vi "ADXL345 I2C Accelerometer.vi"() -> ()   [LabVIEW 2025]
doc: "ADXL345 I2C Accelerometer\n\nThis example shows how to use the ADXL 345 Accelerometer sensor connected to I2C.\n\nThis example expects a USB cable connected from your development PC to the Type B USB Jack (next to the power input) on the roboRIO."
uses:
  <vilib>/Rock Robotics/SystemInterfaces/i2clib/i2c_bus.ctl
  <vilib>/Rock Robotics/WPI/Accelerometer/WPI_AccelerometerADXL345 Axes.ctl
  <vilib>/Rock Robotics/WPI/Accelerometer/ADXL345 Range.ctl
  <vilib>/Rock Robotics/WPI/Accelerometer/WPI_AccelerometerADXL345_I2C_Open.vi
panel:
  out "Z Acceleration":dbl
  out "Y Acceleration":dbl
  in  "Accel Range":T1 items=["+/- 2 g", "+/- 4 g", "+/- 8 g", "+/- 16 g"]
  in  "ADXL345 Axes":T2={"X-Axis"=TRUE, "Y-Axis"=FALSE, "Z-Axis"=FALSE}
  in  "I2C Bus":T3
  out "X Acceleration":dbl
  out "error out":errorcluster
  in  "stop":bool
  # "Set these inputs before running."
  # "Output information"
  # "This shows wiring for the ADXL345 accelerometer on a common sparkfun breakout board."
  # "ADXL345\nGND (black wire)-----\nVCC (red wire)--------\nSCL (yellow wire)-----\nSDA (white wire)------"
  # "roboRIO\nI2C  \nI2C   3.3V\nI2C   SCL\nI2C   SDA"
  # "This shows wiring for the ADXL345 accelerometer on a common kit of parts breakout board.\nNote the I2C header provides 3.3V, so this sensor gets its 5V power from the 5V rail - in this case DIO-0."
  # "ADXL345\n0V (black wire)--------\n5V (red wire)----------\nSCL (yellow wire)-----\nSDA (white wire)------"
  # "roboRIO\nI2C  \nDIO-0  V\nI2C   SCL\nI2C   SDA"
  # "accelerometer"
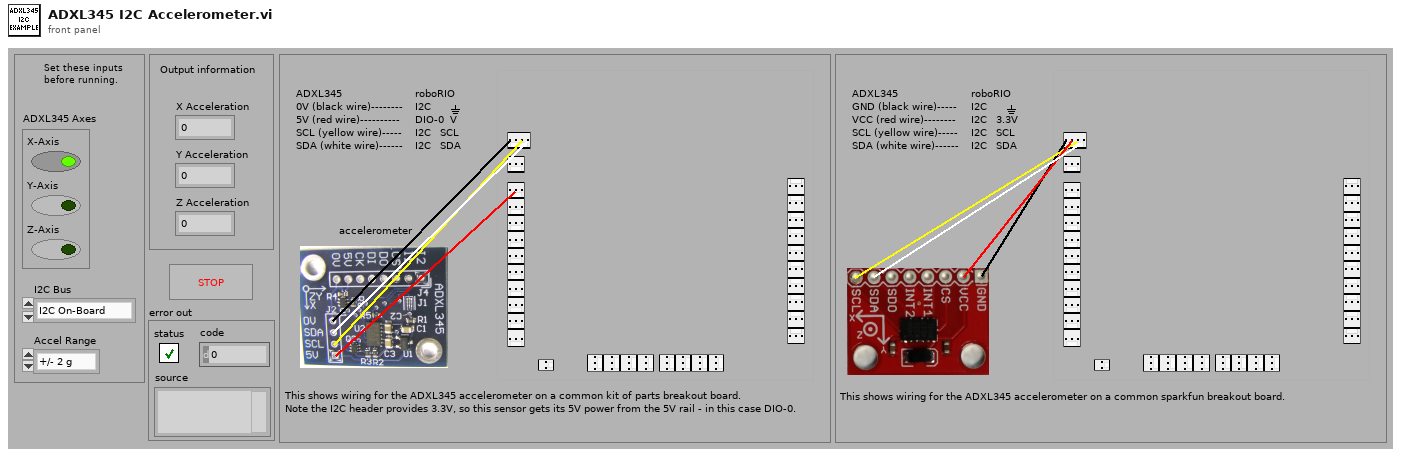
[diagram p1: front panel]
types:
  T1 = typedef "ADXL345 Range.ctl" = u8
  T2 = typedef "WPI_AccelerometerADXL345 Axes.ctl" = cluster{"X-Axis":bool, "Y-Axis":bool, "Z-Axis":bool}
  T3 = typedef "i2c_bus.ctl" = enum16{"I2C On-Board", "I2C MXP", "Invalid"}
  T4 = typedef "WPI_AccelerometerDevRef.ctl" = cluster{"DevStatus":errorcluster, "Scaling":T5, "Analog Channels":T6, "I2C Bus":T3, "SPI Bus":T8, "Accel Range":T1, "ADXL Axes":T2, "Handle":i32, "Device Address":u8, "Accel Type":enum16{"Analog", "ADXL345 I2C", "ADXL345 SPI", "Internal", "ADXL362 SPI"}}
  T5 = typedef "WPI_AccelerometerScaling.ctl" = cluster{"Gain (VoltsPerG)":dbl, "Center Voltage":dbl}
  T6 = typedef "WPI_AccelerometerAnalogChannels.ctl" = cluster{"X-Axis":T7, "Y-Axis":T7, "Z-Axis":T7}
  T7 = typedef "FPGA_AIChannel.ctl" = enum8{"AI 0", "AI 1", "AI 2", "AI 3", "AI MXP 0", "AI MXP 1", "AI MXP 2", "AI MXP 3", "Invalid"}
  T8 = typedef "spi_bus.ctl" = enum16{"SPI On-Board, CS0", "SPI On-Board, CS1", "SPI On-Board, CS2", "SPI On-Board, CS3", "SPI MXP", "Invalid"}
  T9 = cluster{"X-Axis":dbl, "Y-Axis":dbl, "Z-Axis":dbl}
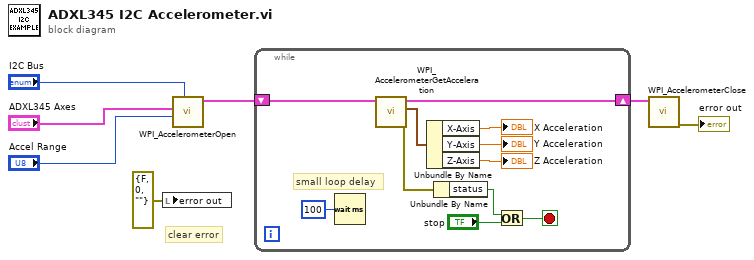
[diagram p0: block diagram]
diagram:
  # "clear error"
  n1 = local write "error out"(errorcluster {"status"=FALSE, "code"=0, "source"=""} ("error out")) -> ()
  n2 = call-poly <vilib>:"WPI_AccelerometerOpen.vi"("I2C Bus"="I2C Bus", "Accel Range"="Accel Range", "ADXL345 Axes"="ADXL345 Axes") -> ("AccelerometerDevRef"=w7:T4)  [unwired: 7 in, 1 out]
  n3 = while {
    shift-right: [w14] -> w2
    shift-left: w7 -> [w12]
    stop <- w13 stop-if-true
    # "small loop delay"
    n4 = Wait (ms)(milliseconds to wait=u32 100) -> ()  [unwired: 1 out]
    n5 = call <vilib>:"WPI_AccelerometerGetAcceleration.vi"("AccelerometerDevRef"=w12) -> ("error out"=w11:errorcluster, "Accelerations"=w15:T9, "AccelerometerDevRef"=w14:T4)  [unwired: 8 in]
    n6 = Unbundle By Name(w15) -> ("X-Axis"=→"X Acceleration":dbl, "Y-Axis"=→"Y Acceleration":dbl, "Z-Axis"=→"Z Acceleration":dbl)
    n7 = Unbundle By Name(w11) -> ("status"=w18:bool)
    n8 = Or(x=w18, y="stop") -> (x .or. y?=w13:bool)
  }
  n9 = call <vilib>:"WPI_AccelerometerClose.vi"("AccelerometerDevRef"=w2) -> ("error out"=→"error out":errorcluster)  [unwired: 10 in]
